vi "Demo.vi"() -> ()   [LabVIEW 2017, in "LT_UpgradeFlash.lvclass"]
uses:
  LT_UpgradeFlash.lvclass
  Global.vi
panel:
  in  "show_btn":bool
  in  "selectChip_btn":bool
  in  "Close_btn":bool
  in  "Open_btn":bool
  in  "Erase_btn":bool
  in  "Read_btn":bool
  in  "chip type":u16(ring)=1 items=["LT9611", "LT6911"]
  in  "Prog_btn":bool
  out "Result String":string
  out "OK?":bool
  in  "burn file path":path=path "D:/Project/Tymphany/LT_UpgradeFlash/HDMI Board/LT FW  Files/LT6911 UXE/lt6911_fw.bin"
  in  "exe path":path=path "D:/Project/Tymphany/LT_UpgradeFlash/HDMI Board/LT Programmer_20240418/LT Programmer.exe"
  in  "Stop Button":bool
  # "操作流程：\n1、选择exe path\n2、\"Open exe\"\n3、选择型号（LT6911/LT9611)，点击\"Select Chip\"\n4、“Erase\""
  # "5、\"Read\"\n6、\"Prog\"\n7、\"Read\""
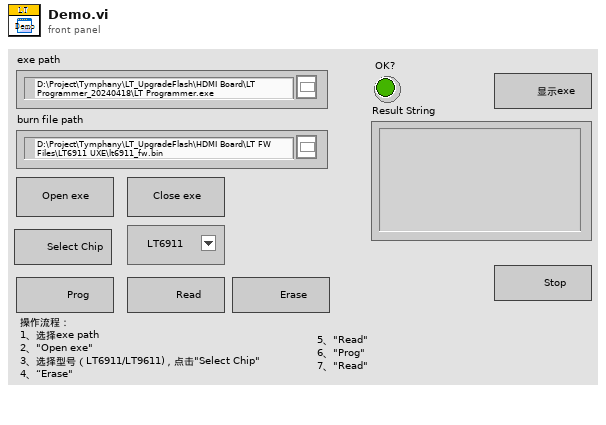
[diagram p1: front panel]
types:
  T1 = enum8{"Enabled", "Disabled", "Disabled and Grayed Out"}
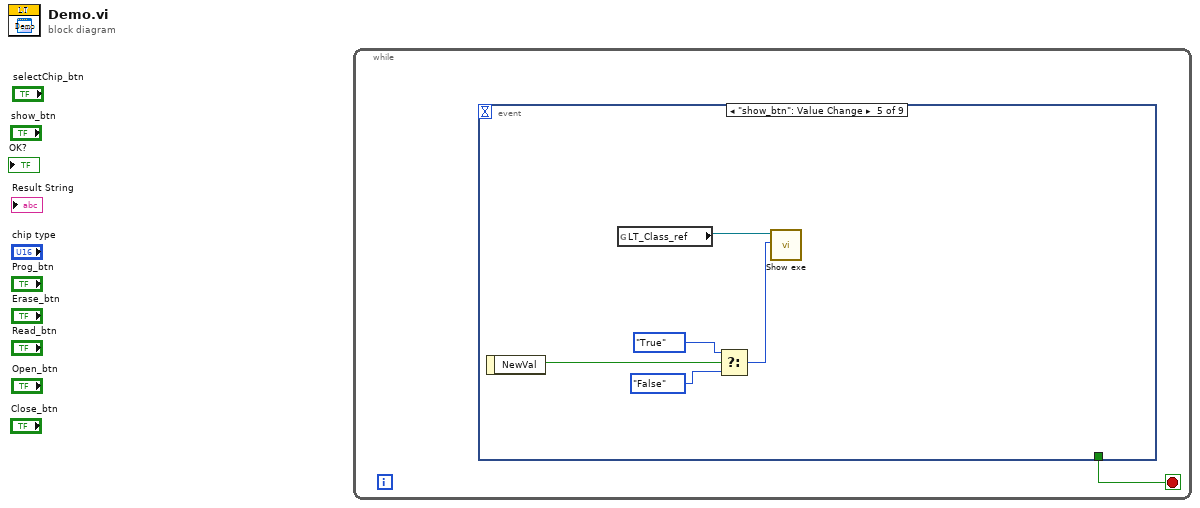
[diagram p0: block diagram]
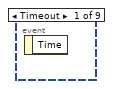
[diagram p2: hidden frame]
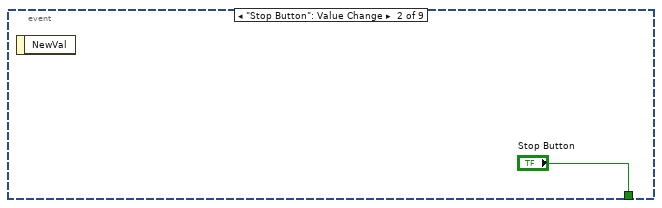
[diagram p3: hidden frame]
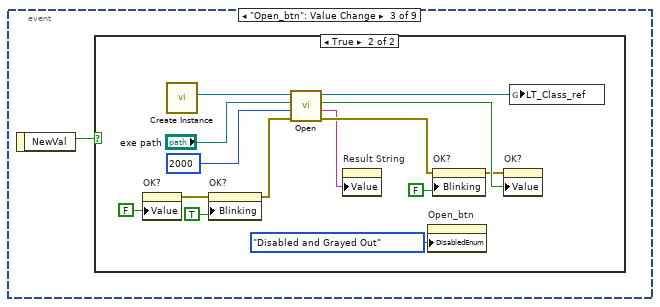
[diagram p4: hidden frame]
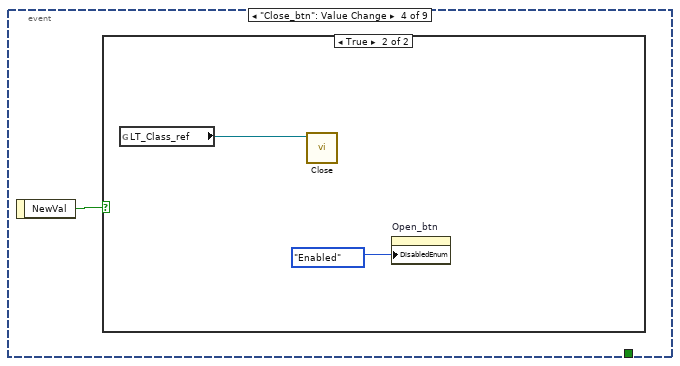
[diagram p6: hidden frame]
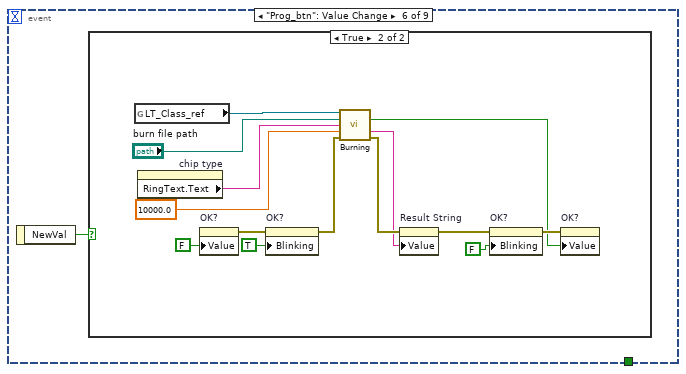
[diagram p8: hidden frame]
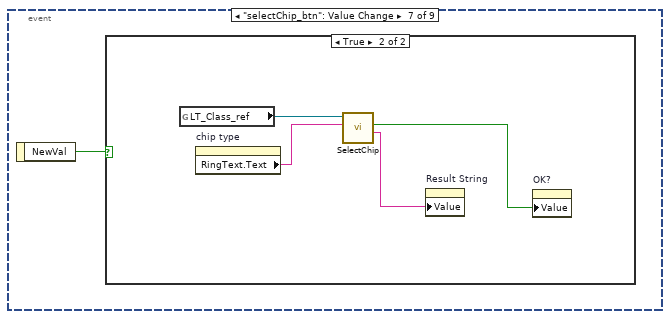
[diagram p10: hidden frame]
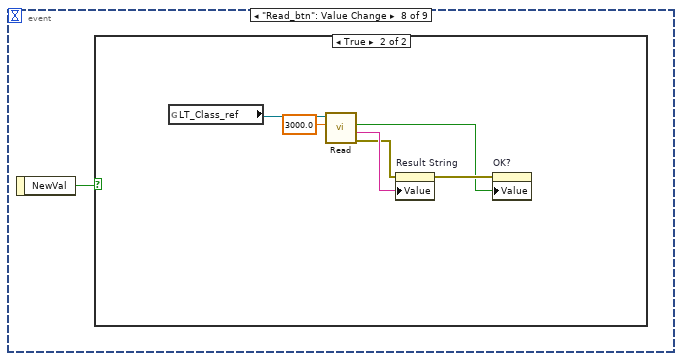
[diagram p12: hidden frame]
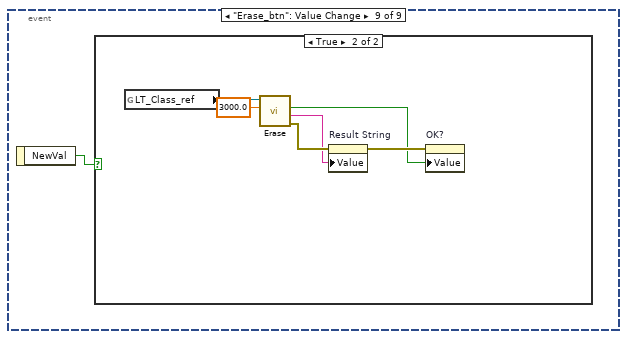
[diagram p14: hidden frame]
diagram:
  n1 = while {
    stop <- w1 stop-if-true
    n2 = event shown="[4] \"show_btn\": Value Change" {
      selector: _ -> [_ _ _ _ _ _ _ _ _]
      dyn-events: _ -> [_ _ _ _ _ _ _ _ _]
      timeout: _ -> [_ _ _ _ _ _ _ _ _]
      tunnel: [_ "Stop Button" _ _ _ _ _ _ _] -> w1
      event Timeout {
        n3 = event-data() -> ()  [unwired: 1 in, 1 out]
      }
      event "Stop Button": Value Change {
        n4 = event-data() -> ()  [unwired: 1 in, 1 out]
      }
      event "Open_btn": Value Change {
        n5 = event-data() -> ("NewVal"=w3:bool)  [unwired: 1 in]
        n6 = case shown="True" w3 {
          frame False {
          }
          frame True {
            n7 = property on="OK?" class="Bool (strict)"("Value"=FALSE ("OK?")) -> (error out=w13:errorcluster)  [unwired: 2 in, 1 out]
            n8 = call "Create Instance.vi"() -> ("LT_UpgradeFlash"=w15:refnum<class "LT_UpgradeFlash.lvclass">)  [unwired: 11 in]
            n9 = property on="OK?" class="Bool (strict)"(error in=w13, "Blinking"=TRUE) -> (error out=w10:errorcluster)  [unwired: 1 in, 1 out]
            n10 = call "Open.vi"("error in (no error)"=w10, "waitForOpenDone(ms)"=2000 ("waitForOpenDone"), "exe path"="exe path", "LT_UpgradeFlash in"=w15) -> ("error out"=w6:errorcluster, "resultStr"=w5:string, "ActionResult"=w8:bool, "LT_UpgradeFlash out"=w14:refnum<class "LT_UpgradeFlash.lvclass">)  [unwired: 4 in]
            n11 = property on="Result String" class="Str"("Value"=w5) -> ()  [unwired: 2 in, 2 out]
            n12 = property on="Open_btn" class="Bool (strict)"("DisabledEnum"=T1."Disabled and Grayed Out" ("Disabled")) -> ()  [unwired: 2 in, 2 out]
            n13 = property on="OK?" class="Bool (strict)"(error in=w6, "Blinking"=FALSE) -> (error out=w7:errorcluster)  [unwired: 1 in, 1 out]
            n14 = property on="OK?" class="Bool (strict)"(error in=w7, "Value"=w8) -> ()  [unwired: 1 in, 2 out]
            n15 = global write "Global.vi" "LT_Class_ref"(w14) -> ()
          }
        }
      }
      event "Close_btn": Value Change {
        n16 = event-data() -> ("NewVal"=w18:bool)  [unwired: 1 in]
        n17 = case shown="True" w18 {
          frame False {
          }
          frame True {
            n18 = global read "Global.vi" "LT_Class_ref"() -> (w20:refnum<class "LT_UpgradeFlash.lvclass">)
            n19 = call "Close.vi"("LT_UpgradeFlash in"=w20) -> ()  [unwired: 9 in, 2 out]
            n20 = property on="Open_btn" class="Bool (strict)"("DisabledEnum"=T1."Enabled" ("Disabled")) -> ()  [unwired: 2 in, 2 out]
          }
        }
      }
      event "show_btn": Value Change {
        n21 = event-data() -> ("NewVal"=w24:bool)  [unwired: 1 in]
        n22 = global read "Global.vi" "LT_Class_ref"() -> (w25:refnum<class "LT_UpgradeFlash.lvclass">)
        n23 = Select(t=enum16{"False", "True"}."True" ("Show"), s=w24, f=enum16{"False", "True"}."False" ("Show")) -> (s? t:f=w21:enum16{"False", "True"})
        n24 = call "Show exe.vi"("Show"=w21, "LT_UpgradeFlash in"=w25) -> ()  [unwired: 8 in, 2 out]
      }
      event "Prog_btn": Value Change {
        n25 = event-data() -> ("NewVal"=w26:bool)  [unwired: 1 in]
        n26 = case shown="True" w26 {
          frame False {
          }
          frame True {
            n27 = global read "Global.vi" "LT_Class_ref"() -> (w40:refnum<class "LT_UpgradeFlash.lvclass">)
            n28 = property on="chip type" class="Ring (strict)"() -> ("RingText.Text"=w27:string)  [unwired: 2 in, 2 out]
            n29 = property on="OK?" class="Bool (strict)"("Value"=FALSE ("OK?")) -> (error out=w38:errorcluster)  [unwired: 2 in, 1 out]
            n30 = property on="OK?" class="Bool (strict)"(error in=w38, "Blinking"=TRUE) -> (error out=w33:errorcluster)  [unwired: 1 in, 1 out]
            n31 = call "Burning.vi"("LT_UpgradeFlash in"=w40, "burnFilePath"="burn file path", "chipName"=w27, "TimeOut(ms)"=10000.0 ("burning time out(ms)"), "error in (no error)"=w33) -> ("ActionResult"=w30:bool, "resultStr"=w31:string, "error out"=w32:errorcluster)  [unwired: 7 in, 1 out]
            n32 = property on="Result String" class="Str"(error in=w32, "Value"=w31) -> (error out=w29:errorcluster)  [unwired: 1 in, 1 out]
            n33 = property on="OK?" class="Bool (strict)"(error in=w29, "Blinking"=FALSE) -> (error out=w37:errorcluster)  [unwired: 1 in, 1 out]
            n34 = property on="OK?" class="Bool (strict)"(error in=w37, "Value"=w30) -> ()  [unwired: 1 in, 2 out]
          }
        }
      }
      event "selectChip_btn": Value Change {
        n35 = event-data() -> ("NewVal"=w41:bool)  [unwired: 1 in]
        n36 = case shown="True" w41 {
          frame False {
          }
          frame True {
            n37 = global read "Global.vi" "LT_Class_ref"() -> (w45:refnum<class "LT_UpgradeFlash.lvclass">)
            n38 = property on="chip type" class="Ring (strict)"() -> ("RingText.Text"=w44:string)  [unwired: 2 in, 2 out]
            n39 = call "SelectChip.vi"("chipSelection"=w44, "LT_UpgradeFlash in"=w45) -> ("resultStr"=w43:string, "ActionResult"=w42:bool)  [unwired: 6 in, 2 out]
            n40 = property on="Result String" class="Str"("Value"=w43) -> ()  [unwired: 2 in, 2 out]
            n41 = property on="OK?" class="Bool (strict)"("Value"=w42) -> ()  [unwired: 2 in, 2 out]
          }
        }
      }
      event "Read_btn": Value Change {
        n42 = event-data() -> ("NewVal"=w46:bool)  [unwired: 1 in]
        n43 = case shown="True" w46 {
          frame False {
          }
          frame True {
            n44 = global read "Global.vi" "LT_Class_ref"() -> (w52:refnum<class "LT_UpgradeFlash.lvclass">)
            n45 = call "Read.vi"("TimeOut(s)"=3000.0, "LT_UpgradeFlash in"=w52) -> ("error out"=w49:errorcluster, "resultStr"=w50:string, "ActionResult"=w48:bool)  [unwired: 6 in, 1 out]
            n46 = property on="Result String" class="Str"(error in=w49, "Value"=w50) -> (error out=w51:errorcluster)  [unwired: 1 in, 1 out]
            n47 = property on="OK?" class="Bool (strict)"(error in=w51, "Value"=w48) -> ()  [unwired: 1 in, 2 out]
          }
        }
      }
      event "Erase_btn": Value Change {
        n48 = event-data() -> ("NewVal"=w53:bool)  [unwired: 1 in]
        n49 = case shown="True" w53 {
          frame False {
          }
          frame True {
            n50 = global read "Global.vi" "LT_Class_ref"() -> (w59:refnum<class "LT_UpgradeFlash.lvclass">)
            n51 = call "Erase.vi"("timeOut(ms)"=3000.0, "LT_UpgradeFlash in"=w59) -> ("error out"=w57:errorcluster, "resultStr"=w56:string, "ActionResult"=w55:bool)  [unwired: 6 in, 1 out]
            n52 = property on="Result String" class="Str"(error in=w57, "Value"=w56) -> (error out=w58:errorcluster)  [unwired: 1 in, 1 out]
            n53 = property on="OK?" class="Bool (strict)"(error in=w58, "Value"=w55) -> ()  [unwired: 1 in, 2 out]
          }
        }
      }
    }
  }
